vi "Error_3.vi"(7 "Current PNG filename":string, 8 "error in (no error)":errorcluster, 10 "Standard error":string, 11 "C return":i32) -> (0 "error out":errorcluster, 2 "Standard error":string)   [LabVIEW 2023]
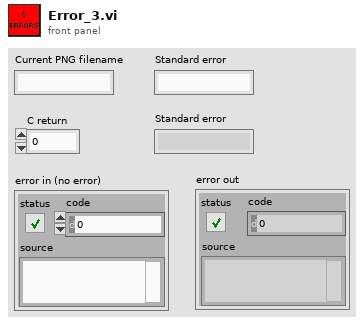
[diagram p1: front panel]
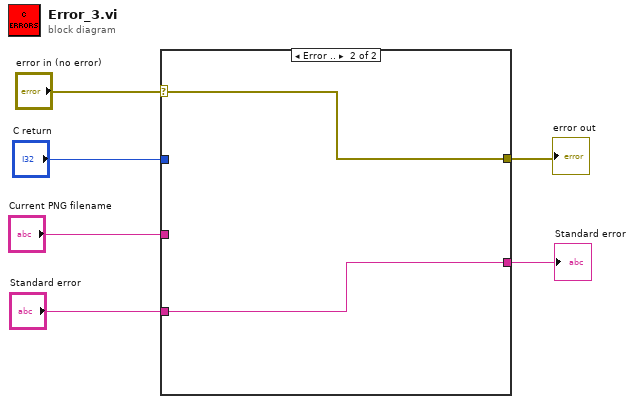
[diagram p0: block diagram]
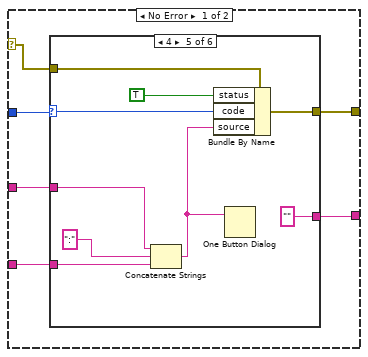
[diagram p2: hidden frame]
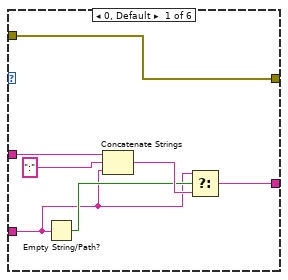
[diagram p3: hidden frame]
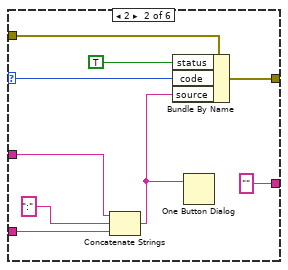
[diagram p4: hidden frame]
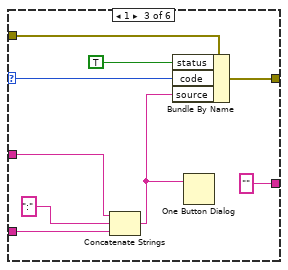
[diagram p5: hidden frame]
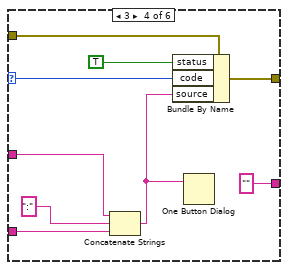
[diagram p6: hidden frame]
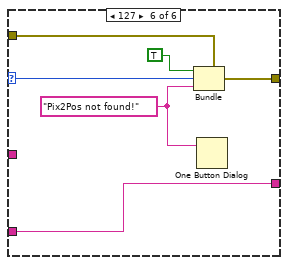
[diagram p7: hidden frame]
diagram:
  n1 = case shown="Error .." "error in (no error)" {
    selector: "error in (no error)" -> [w11 w63]
    tunnel: "C return" -> [w12 _]
    tunnel: "Current PNG filename" -> [w9 _]
    tunnel: "Standard error" -> [w10 w62]
    tunnel: [w8 w63] -> w2
    tunnel: [w7 w62] -> w1
    frame No Error {
      n2 = case shown="4" w12 {
        selector: w12 -> [_ w26 w35 w44 w53 w60]
        tunnel: w11 -> [w19 w28 w37 w46 w55 w61]
        tunnel: w10 -> [w13 w25 w34 w43 w52 w56]
        tunnel: w9 -> [w18 w23 w32 w41 w50 _]
        tunnel: [w19 w21 w30 w39 w48 w58] -> w8
        tunnel: [w14 "" "" "" "" w56] -> w7
        frame 0, Default {
          n3 = Empty String/Path?(string/path=w13) -> (empty?=w15:bool)
          n4 = Concatenate Strings(w18, ":", w13) -> (w16:string)
          n5 = Select(t=w13, s=w15, f=w16) -> (s? t:f=w14:string)
        }
        frame 2 {
          n6 = Concatenate Strings(w23, ":", w25) -> (w22:string)
          n7 = Bundle By Name(cluster=w28, "status"=TRUE, "code"=w26, "source"=w22) -> (w21:errorcluster)
          n8 = One Button Dialog(message=w22) -> ()  [unwired: 1 in, 1 out]
        }
        frame 1 {
          n9 = Concatenate Strings(w32, ":", w34) -> (w31:string)
          n10 = Bundle By Name(cluster=w37, "status"=TRUE, "code"=w35, "source"=w31) -> (w30:errorcluster)
          n11 = One Button Dialog(message=w31) -> ()  [unwired: 1 in, 1 out]
        }
        frame 3 {
          n12 = Concatenate Strings(w41, ":", w43) -> (w40:string)
          n13 = Bundle By Name(cluster=w46, "status"=TRUE, "code"=w44, "source"=w40) -> (w39:errorcluster)
          n14 = One Button Dialog(message=w40) -> ()  [unwired: 1 in, 1 out]
        }
        frame 4 {
          n15 = Concatenate Strings(w50, ":", w52) -> (w49:string)
          n16 = Bundle By Name(cluster=w55, "status"=TRUE, "code"=w53, "source"=w49) -> (w48:errorcluster)
          n17 = One Button Dialog(message=w49) -> ()  [unwired: 1 in, 1 out]
        }
        frame 127 {
          w57 = "Pix2Pos not found!"
          n18 = Bundle(cluster=w61, "status"=TRUE, "code"=w60, "source"=w57) -> (w58:errorcluster)
          n19 = One Button Dialog(message=w57) -> ()  [unwired: 1 in, 1 out]
        }
      }
    }
    frame Error {
    }
  }
  "Standard error" <- w1
  "error out" <- w2
